vi "AFM_Driver_Manager.CloseVIReferences.vi"(8 "error in (no error)":errorcluster, 11 "AFM_Driver_Manager in":refnum<class "AFM_Driver_Manager.lvclass">) -> (0 "error out":errorcluster, 3 "AFM_Driver_Manager out":refnum<class "AFM_Driver_Manager.lvclass">)   [LabVIEW 2019, in "AFM_Driver_Manager.lvclass"]
uses:
  AFM_Driver_Manager.lvclass
  AFM_Driver_Manager.lvclass/AFM_Driver_Manager.ctl
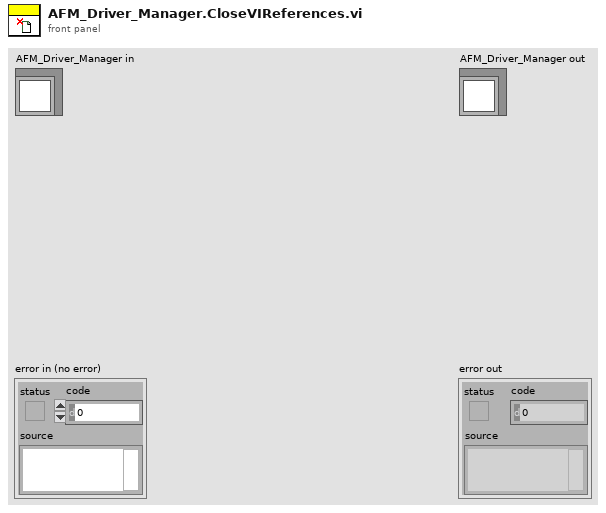
[diagram p1: front panel]
types:
  T1 = typedef "AFM_Driver_Manager.lvclass/AFM_Driver_Manager.PublicMethods.ctl" = cluster{"Stop Event":refnum<user-event>, "Lithography Data":refnum<user-event>, "Run Lithography":refnum<user-event>, "Background Image":refnum<user-event>, "Abort Notifier":refnum<user-event>}
  T2 = cluster{"VI Refnum":refnum<vi>, "Path":path, "Name":string, "Events":T1}[]
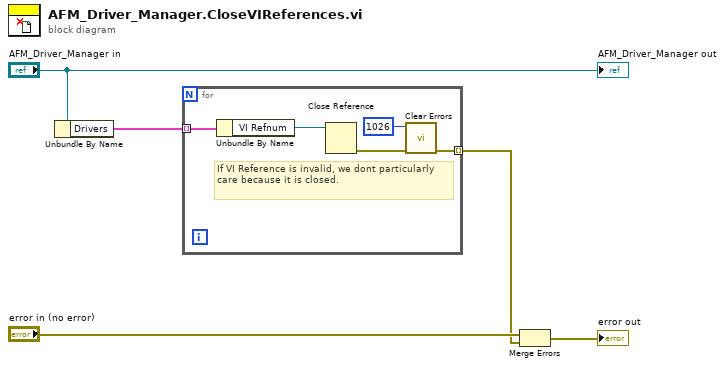
[diagram p0: block diagram]
diagram:
  n1 = Unbundle By Name("AFM_Driver_Manager in") -> ("Drivers"=w3:T2)
  n2 = for {
    tunnel: w3 -> [w10] mode=indexing
    tunnel: [w7] -> w2 mode=indexing
    # "If VI Reference is invalid, we dont particularly care because it is closed."
    n3 = Unbundle By Name(w10) -> ("VI Refnum"=w9:refnum<vi>)
    n4 = Close Reference(reference=w9) -> (error out=w8:errorcluster)  [unwired: 1 in]
    n5 = call <vilib>:"Clear Errors.vi"("error in (no error)"=w8, "specific error code to clear (0: all)"=1026) -> ("error out"=w7:errorcluster)  [unwired: 4 in, 1 out]
  }
  n6 = Merge Errors("error in (no error)", w2) -> (→"error out":errorcluster)
  "AFM_Driver_Manager out" <- "AFM_Driver_Manager in"
